vi "LINC Get ID Info.vi"(8 "error in (no error)":errorcluster, 10 "mode (CMD)":enum16{"CMD", "TLM"}(ring), 11 "LINC session":refnum<class "LINC.lvclass">) -> (0 "error out":errorcluster, 1 "bit size":i32, 2 "bit offset":i32, 3 "dup LINC session":refnum<class "LINC.lvclass">, 4 "IDs":i32[](array[numeric]))   [LabVIEW 2018, in "STEPkgDriver_LINC.lvlib" / "LINC.lvclass"]
uses:
  LINC.lvclass
  STEPkgDriver_LINC.lvlib
  LINC Global Mode.ctl
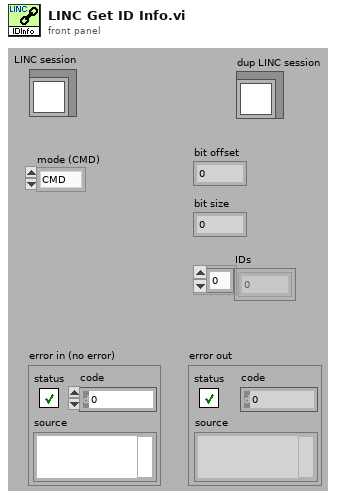
[diagram p1: front panel]
types:
  T1 = typedef "STEPkgDriver_LINC.lvlib/LINC Global Mode.ctl" = enum16{"INIT", "CLEAR", "ADD_PKT_HDR", "ADD_PKT", "GET_PKT_NAMES", "GET_PKT_DESC", "GET_PKT_HDR", "GET_PKT", "SET_PKT", "SET_DATA", "SIM_EN", "SIM_DS"}
  T2 = typedef "STEPkgDriver_LINC.lvlib/LINC Format Prototype.ctl" = cluster{"type":string, "bit offset":i32, "bit size":i32, "format":string, "unit":string, "description":string, "state values":i64[], "states":string[], "max":string, "min":string, "default":string, "array":bool, "bit element size":i32, "poly bound":dbl[], "poly scale":cluster{"coefficients":dbl[]}[], "labview size":i32, "simulate":bool, "ID":bool, "required":bool}
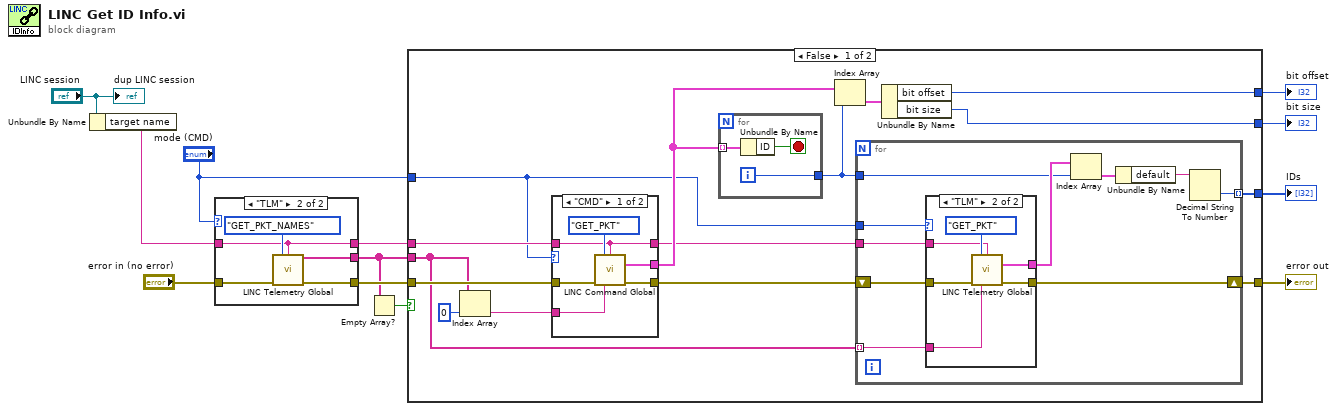
[diagram p0: block diagram]
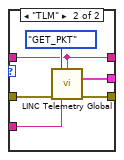
[diagram p2: hidden frame]
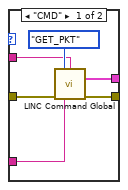
[diagram p3: hidden frame]
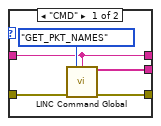
[diagram p5: hidden frame]
diagram:
  n1 = Unbundle By Name("LINC session") -> ("target name"=w10:string)
  n2 = case shown="\"TLM\"" "mode (CMD)" {
    tunnel: [w16 w21] -> w12
    tunnel: [w15 w20] -> w2
    tunnel: w10 -> [w13 w18]
    tunnel: "error in (no error)" -> [w14 w19]
    tunnel: [w13 w18] -> w6
    frame "CMD" {
      n3 = call "LINC Command Global.vi"("mode"=LINC_Global_Mode."GET_PKT_NAMES", "target name"=w13, "error in (no error)"=w14) -> ("values out"=w15:string[], "error out"=w16:errorcluster)  [unwired: 8 in, 3 out]
    }
    frame "TLM" {
      n4 = call "LINC Telemetry Global.vi"("mode"=LINC_Global_Mode."GET_PKT_NAMES", "target name"=w18, "error in (no error)"=w19) -> ("values out"=w20:string[], "error out"=w21:errorcluster)  [unwired: 8 in, 3 out]
    }
  }
  n5 = Empty Array?(array=w2) -> (empty?=w1:bool)
  n6 = case shown="False" w1 {
    tunnel: w12 -> [w36 w75]
    tunnel: w2 -> [w33 _]
    tunnel: [w32 _] -> w11
    tunnel: [w29 w75] -> w9
    tunnel: w6 -> [w28 _]
    tunnel: "mode (CMD)" -> [w26 _]
    tunnel: [w24 _] -> w4
    tunnel: [w23 _] -> w3
    frame False {
      n7 = Index Array(array=w33, index=0) -> (element=w25:string)
      n8 = case shown="\"CMD\"" w26 {
        tunnel: w36 -> [w42 w48]
        tunnel: [w41 w47] -> w31
        tunnel: [w40 w46] -> w30
        tunnel: w28 -> [w39 w45]
        tunnel: [w39 w45] -> w27
        tunnel: w25 -> [w38 w44]
        frame "CMD" {
          n9 = call "LINC Command Global.vi"("mode"=LINC_Global_Mode."GET_PKT", "target name"=w39, "error in (no error)"=w42, "packet name"=w38) -> ("item formats out"=w41:T2[], "error out"=w40:errorcluster)  [unwired: 7 in, 3 out]
        }
        frame "TLM" {
          n10 = call "LINC Telemetry Global.vi"("mode"=LINC_Global_Mode."GET_PKT", "target name"=w45, "error in (no error)"=w48, "packet name"=w44) -> ("item formats out"=w47:T2[], "error out"=w46:errorcluster)  [unwired: 7 in, 3 out]
        }
      }
      n11 = for {
        tunnel: w31 -> [w74] mode=indexing
        tunnel: [w72] -> w34
        i -> [w72]
        stop <- w73 stop-if-true
        n12 = Unbundle By Name(w74) -> ("ID"=w73:bool)
      }
      n13 = Index Array(array=w31, index=w34) -> (element=w37:T2)
      n14 = for {
        tunnel: w34 -> [w55]
        tunnel: w33 -> [w50] mode=indexing
        shift-right: [w58] -> w29
        shift-left: w30 -> [w59]
        tunnel: w27 -> [w57]
        tunnel: [w52] -> w32 mode=indexing
        tunnel: w26 -> [w51]
        n15 = case shown="\"TLM\"" w51 {
          tunnel: w59 -> [w64 w70]
          tunnel: [w63 w69] -> w58
          tunnel: w57 -> [w62 w68]
          tunnel: [w61 w67] -> w56
          tunnel: w50 -> [w60 w66]
          frame "CMD" {
            n16 = call "LINC Command Global.vi"("mode"=LINC_Global_Mode."GET_PKT", "target name"=w62, "error in (no error)"=w64, "packet name"=w60) -> ("item formats out"=w61:T2[], "error out"=w63:errorcluster)  [unwired: 7 in, 3 out]
          }
          frame "TLM" {
            n17 = call "LINC Telemetry Global.vi"("mode"=LINC_Global_Mode."GET_PKT", "target name"=w68, "error in (no error)"=w70, "packet name"=w66) -> ("item formats out"=w67:T2[], "error out"=w69:errorcluster)  [unwired: 7 in, 3 out]
          }
        }
        n18 = Index Array(array=w56, index=w55) -> (element=w54:T2)
        n19 = Unbundle By Name(w54) -> ("default"=w53:string)
        n20 = Decimal String To Number(string=w53) -> (number=w52:i32)  [unwired: 2 in, 1 out]
      }
      n21 = Unbundle By Name(w37) -> ("bit offset"=w24:i32, "bit size"=w23:i32)
    }
    frame True {
    }
  }
  "error out" <- w9
  "bit offset" <- w4
  "bit size" <- w3
  "IDs" <- w11
  "dup LINC session" <- "LINC session"
